vi "End.vi"(8 "error in (no error)":errorcluster, 11 "Channel in":refnum<class "Channel.lvclass">) -> (0 "error out":errorcluster, 3 "Channel out":refnum<class "Channel.lvclass">)   [LabVIEW 2018, in "Channel.lvclass"]
doc: "End the ACS execution \n\nThis function is responsible for eding the ACS execution correctly"
uses:
  Channel.lvclass
  Channel.lvclass/Channel.ctl
  Simulated_CCD_Camera/Simulated Camera.lvclass
  Header content/Header content.lvclass
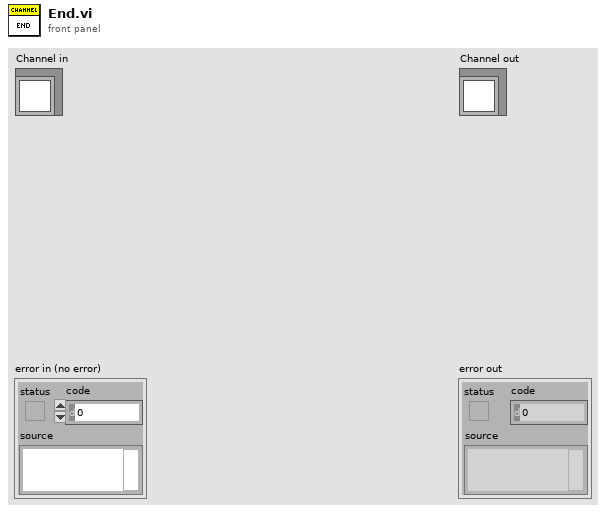
[diagram p1: front panel]
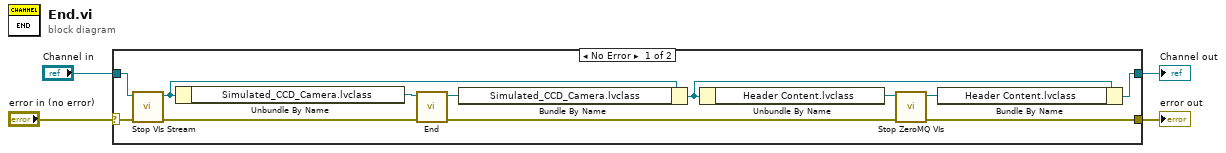
[diagram p0: block diagram]
diagram:
  n1 = case shown="No Error" "error in (no error)" {
    selector: "error in (no error)" -> [w13 w18]
    tunnel: [w6 w18] -> w3
    tunnel: [w9 w17] -> w1
    tunnel: "Channel in" -> [w16 w17]
    frame No Error {
      n2 = call "Stop VIs Stream.vi"("error in (no error)"=w13, "Channel in"=w16) -> ("error out"=w11:errorcluster, "Channel out"=w12:refnum<class "Channel.lvclass">)  [unwired: 8 in]
      n3 = Unbundle By Name(w12) -> ("Simulated_CCD_Camera.lvclass"=w15:refnum<class "Simulated Camera.lvclass">)
      n4 = call "End.vi"("error in (no error)"=w11, "Simulated_CCD_Camera in"=w15) -> ("error out"=w5:errorcluster, "Simulated_CCD_Camera out"=w14:refnum<class "Simulated Camera.lvclass">)  [unwired: 8 in]
      n5 = Bundle By Name(cluster=w12, "Simulated_CCD_Camera.lvclass"=w14) -> (w10:refnum<class "Channel.lvclass">)
      n6 = Unbundle By Name(w10) -> ("Header Content.lvclass"=w8:refnum<class "Header content.lvclass">)
      n7 = call "Stop ZeroMQ VIs.vi"("error in (no error)"=w5, "Header content in"=w8) -> ("error out"=w6:errorcluster, "Header content out"=w7:refnum<class "Header content.lvclass">)  [unwired: 8 in]
      n8 = Bundle By Name(cluster=w10, "Header Content.lvclass"=w7) -> (w9:refnum<class "Channel.lvclass">)
    }
    frame Error {
    }
  }
  "error out" <- w3
  "Channel out" <- w1
